vi "Autonomous Globals.vi"() -> ()   [LabVIEW 2017]
panel:
  in  "Auto Cals":dbl[](array[numeric])
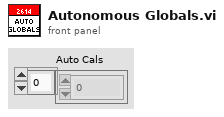
[diagram p1: front panel]
diagram:
